vi "Test_Pre_Loop_Initialization_FGV.vi"(8 "error in (no error)":errorcluster, 10 "DUT":string, 11 "VI in":refnum<vi>) -> (0 "error out":errorcluster, 2 "queue out":refnum<queue>, 3 "User Event out":refnum<user-event>)   [LabVIEW 2024, in "Test_2.lvlib"]
doc: "This VI\n------------------------------------------------\nPer_Loop_Initialize\n------------------------------------------------\n-Generate the Communication Queue Reference with FGV.\n-Get the Common User Events Reference at Application Level."
uses:
  Test_2.lvlib
  PrivateControls/Test_FGV_Queue_Control.ctl
  UserEvents/Controls/User_Events_Action_Control.ctl
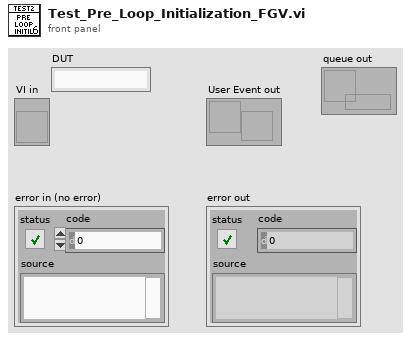
[diagram p1: front panel]
types:
  T1 = typedef "Test_2.lvlib/User_Events_Action_Control.ctl" = enum16{"Get", "Create", "Destroy"}
  T2 = cluster{"Message":string, "Message Data":variant}
  T3 = typedef "Test_2.lvlib/Test_FGV_Queue_Control.ctl" = enum16{"Release", "Get", "Set", "Flush"}
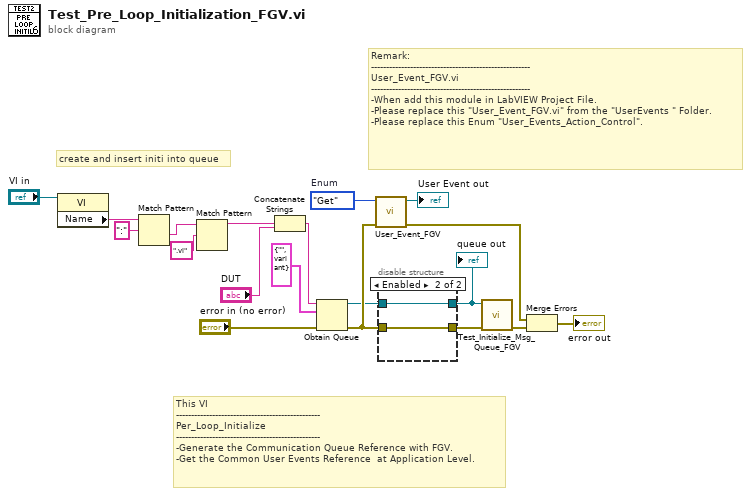
[diagram p0: block diagram]
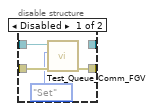
[diagram p2: hidden frame]
diagram:
  w14 = User_Events_Action_Control."Get"  # Enum
  # "Remark:\n-----------------------------------------------------\nUser_Event_FGV.vi\n-----------------------------------------------------\n-When add this module in LabVIEW Project File.\n-Please replace this \"User_Event_FGV.vi\" from the \"UserEvents \" Folder.\n-Please replace this Enum \"User_Events_Action_Control\"."
  # "This VI\n------------------------------------------------\nPer_Loop_Initialize\n------------------------------------------------\n-Generate the Communication Queue Reference with FGV.\n-Get the Common User Events Reference  at Application Level."
  # "create and insert initi into queue"
  n1 = property class="VI"(reference="VI in") -> ("Name"=w6:string)  [unwired: 1 in, 2 out]
  n2 = Match Pattern(string=w6, regular expression=":") -> (after substring=w3:string)  [unwired: 1 in, 3 out]
  n3 = Match Pattern(string=w3, regular expression=".vi") -> (before substring=w2:string)  [unwired: 1 in, 3 out]
  n4 = Concatenate Strings(w2, "DUT") -> (w8:string)
  n5 = Obtain Queue(name (unnamed)=w8, element data type=T2 {"Message"="", "Message Data"=variant} ("Message Cluster"), error in (no error)="error in (no error)") -> (queue out=w13:refnum<queue>, error out=w15:errorcluster)  [unwired: 2 in, 1 out]
  n6 = call "User_Event_FGV.vi"("error in (no error)"=w15, "Enum"=w14) -> ("error out"=w17:errorcluster, "User Event out"=→"User Event out":refnum<user-event>)  [unwired: 8 in]
  n7 = disable-structure shown="Enabled" {
    disable-tunnel: w15 -> [w23 w24]
    disable-tunnel: w13 -> [w22 w25]
    disable-tunnel: [w21 w24] -> w11
    disable-tunnel: [_ w25] -> w4
    frame Disabled {
      n8 = call "Test_Queue_Comm_FGV.vi"("error in (no error)"=w23, "Enum"=Test_FGV_Queue_Control."Set", "queue in"=w22) -> ("error Out"=w21:errorcluster)  [unwired: 7 in, 1 out]
    }
    frame Enabled {
    }
  }
  "queue out" <- w4
  n9 = call "Test_Initialize_Msg_Queue_FGV.vi"("error in (no error)"=w11, "queue in"=w4) -> ("error out"=w18:errorcluster)  [unwired: 9 in]
  n10 = Merge Errors(w17, w18) -> (→"error out":errorcluster)
